vi "Calibration.vi"(2 "Analogue In":refnum<k21>, 3 "Digital In":refnum<k21>) -> (0 "Analogue In Out":refnum<k21>, 1 "Digital Out":refnum<k21>)   [LabVIEW 2015]
uses:
  CalibrationEnum.ctl
  <vilib>/DAQmx/write.llb/DAQmx Write (Digital 1D Bool NChan 1Samp 1Line).vi
  <vilib>/DAQmx/write.llb/DAQmx Write (Analog 1D DBL NChan 1Samp).vi
  GlobalVariables.vi
  <vilib>/DAQmx/create/channels.llb/DAQmx Create Channel (AO-Voltage-Basic).vi
  <vilib>/DAQmx/create/channels.llb/DAQmx Create Channel (DO-Digital Output).vi
  <vilib>/DAQmx/miscellaneous.llb/DAQmx Fill In Error Info.vi
  <resource>/objmgr/daqmx.rc
panel:
  in  "Listbox":i32(listbox)
  in  "Calibration Coordinates":T1
  in  "Calibration Map":T2
  in  "Piezo Focus /um":dbl(slide)=5.0 scale=0.0..10.0
  out "Enum":T3=enum."YMirrorVolt"
  in  "stop":bool
  in  "Z Voltage /V":dbl(slide)=-3.815028901734104 scale=-10.0..10.0
  in  "Y Voltage /V":dbl(slide)=2.485549132947977 scale=-10.0..10.0
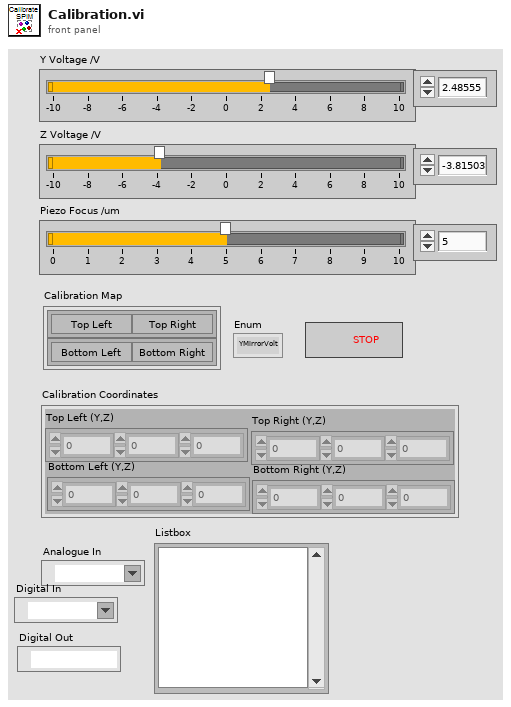
[diagram p1: front panel]
types:
  T1 = cluster{"Top Left (Y,Z)":dbl[], "Top Right (Y,Z)":dbl[], "Bottom Left (Y,Z)":dbl[], "Bottom Right (Y,Z)":dbl[]}
  T2 = cluster{"Cluster 2":cluster{"Top Left":bool, "Top Right":bool}, "Cluster":cluster{"Bottom Left":bool, "Bottom Right":bool}}
  T3 = typedef "CalibrationEnum.ctl" = enum16{"PiezoVolt", "YMirrorVolt", "ZMirrorVolt", "idle"}
  T4 = cluster{dbl[], "Top Right (Y,Z)":dbl[], "Bottom Left (Y,Z)":dbl[], "Bottom Right (Y,Z)":dbl[]}
  T5 = cluster{"Top Left (Y,Z)":dbl[], dbl[], "Bottom Left (Y,Z)":dbl[], "Bottom Right (Y,Z)":dbl[]}
  T6 = cluster{"Top Left (Y,Z)":dbl[], "Top Right (Y,Z)":dbl[], dbl[], "Bottom Right (Y,Z)":dbl[]}
  T7 = cluster{"Top Left (Y,Z)":dbl[], "Top Right (Y,Z)":dbl[], "Bottom Left (Y,Z)":dbl[], dbl[]}
  T8 = cluster{"Top Left":dbl[], "Top Right":dbl[], "Bottom Left":dbl[], "Bottom Right":dbl[]}
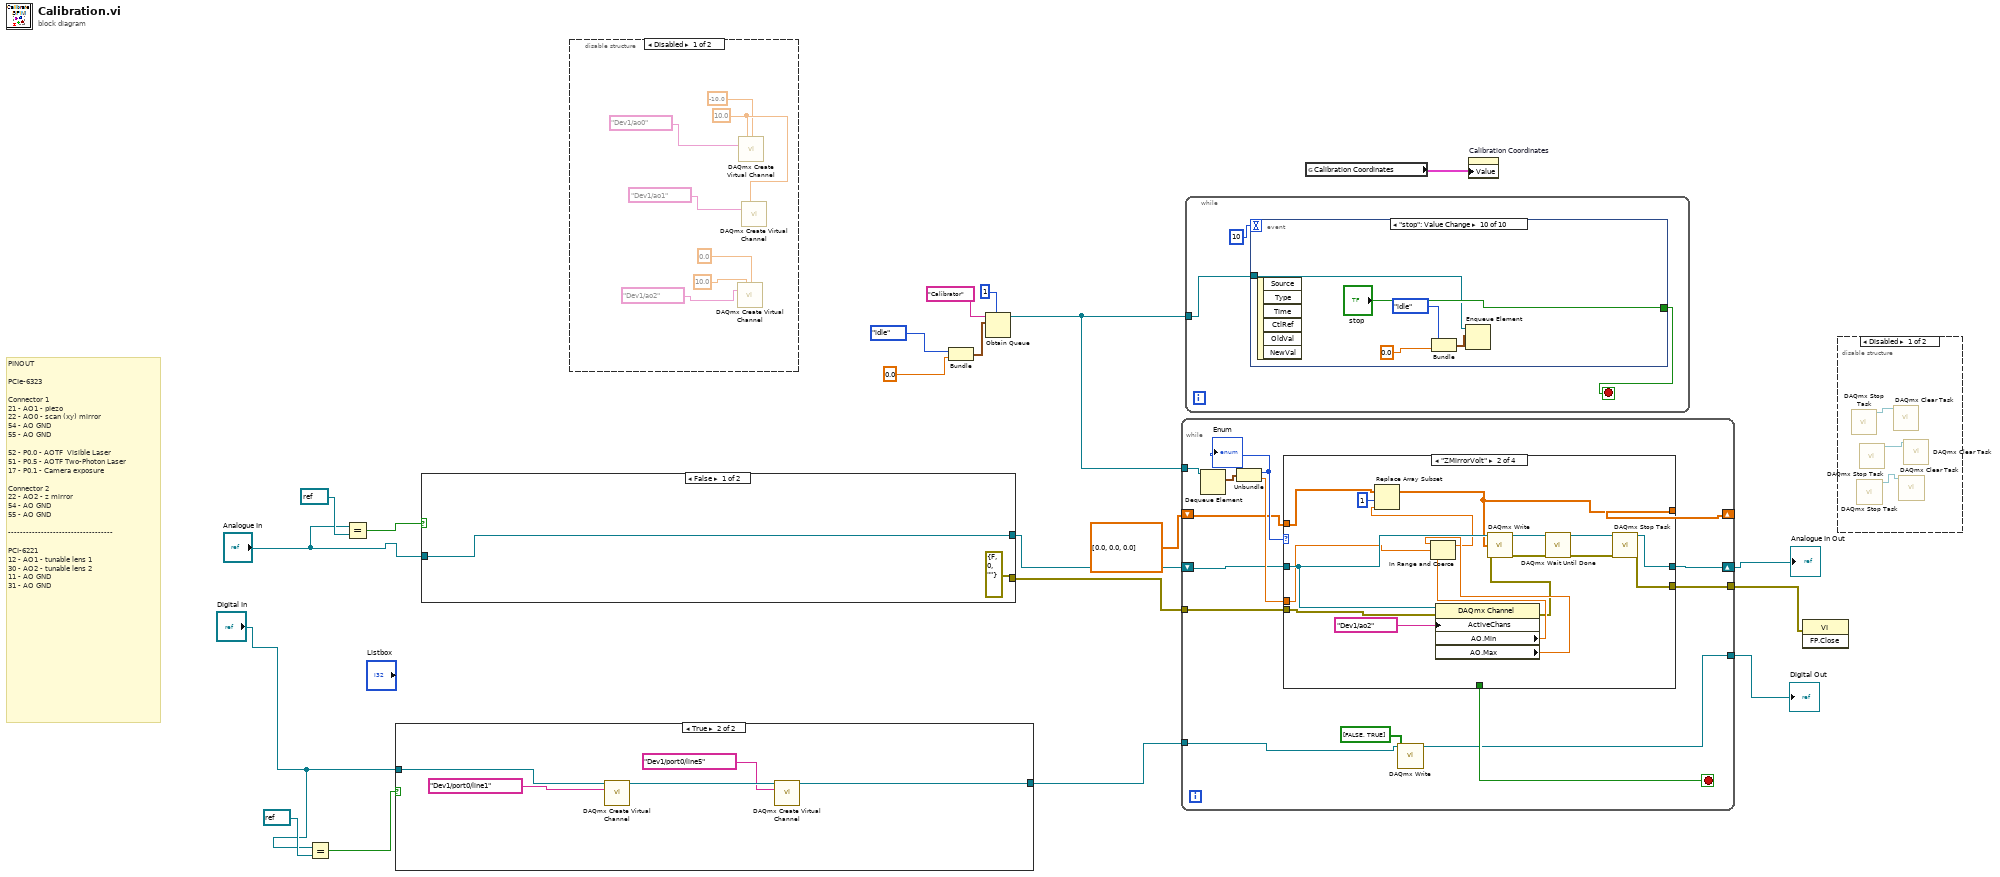
[diagram p0: block diagram]
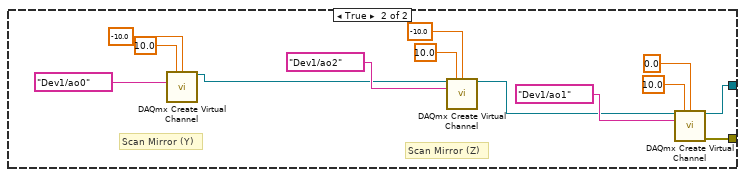
[diagram p3: hidden frame]
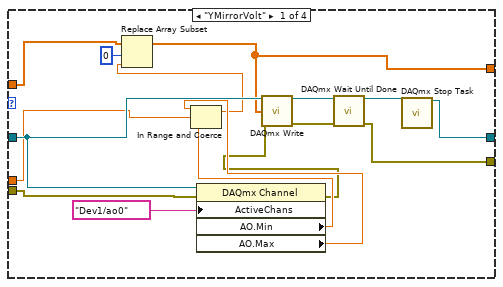
[diagram p6: hidden frame]
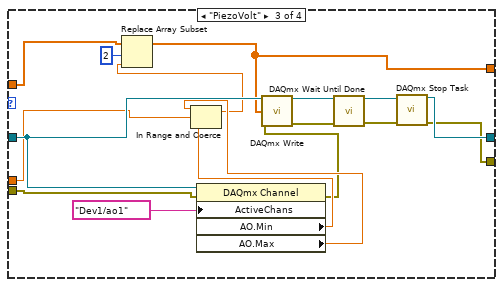
[diagram p7: hidden frame]
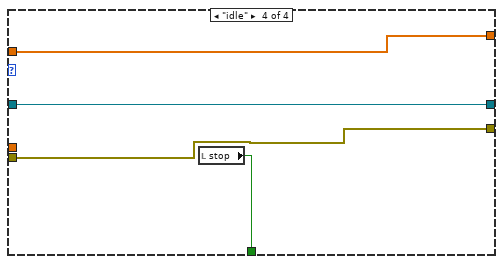
[diagram p8: hidden frame]
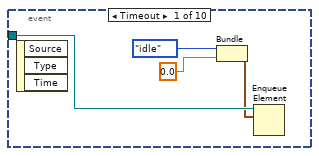
[diagram p9: hidden frame]
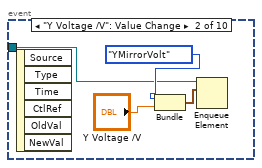
[diagram p10: hidden frame]
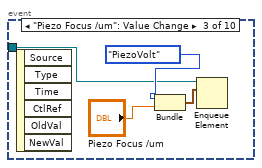
[diagram p11: hidden frame]
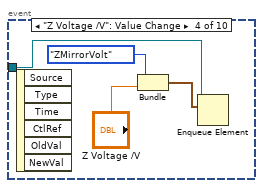
[diagram p12: hidden frame]
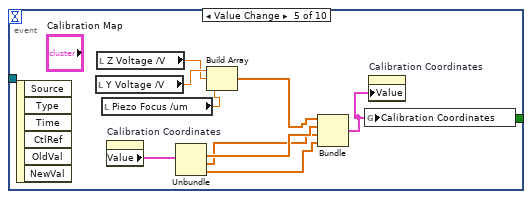
[diagram p13: hidden frame]
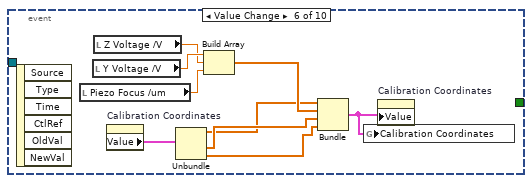
[diagram p14: hidden frame]
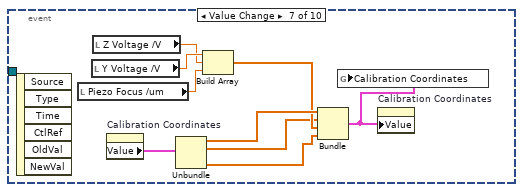
[diagram p15: hidden frame]
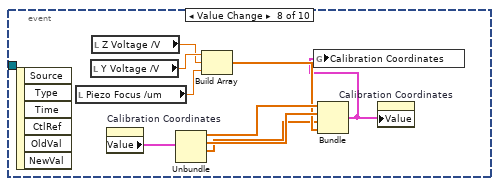
[diagram p16: hidden frame]
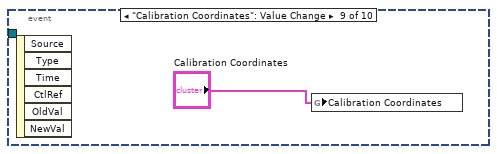
[diagram p17: hidden frame]
diagram:
  # "PINOUT\n\nPCIe-6323\n\nConnector 1\n21 - AO1 - piezo\n22 - AO0 - scan (xy) mirror\n54 - AO GND\n55 - AO GND\n\n52 - P0.0 - AOTF  Visible Laser\n51 - P0.5 - AOTF Two-Photon Laser\n17 - P0.1 - Camera exposure\n\nConnector 2\n22 - AO2 - z mirror\n54 - AO GND\n55 - AO GND\n\n-----------------------------------\n\nPCI-6221\n12 - AO1 - tunable lens 1\n30 - AO2 - tunable lens 2\n11 - AO GND\n31 - AO GND"
  n1 = Equal?(x="Digital In", y=refnum<k21> refnum ("Mirror Y")) -> (x = y?=w2:bool)
  n2 = Equal?(x="Analogue In", y=refnum<k21> refnum ("Mirror Y")) -> (x = y?=w12:bool)
  n3 = case shown="True" w2 {
    tunnel: "Digital In" -> [w21 w23]
    tunnel: [w21 w22] -> w1
    frame False {
    }
    frame True {
      n4 = call-poly <vilib>:"DAQmx Create Virtual Channel.vi"("task in"=w23, "lines"=tag "Dev1/port0/line1") -> ("task out"=w26:refnum<k21>)  [unwired: 12 in, 1 out]
      n5 = call-poly <vilib>:"DAQmx Create Virtual Channel.vi"("task in"=w26, "lines"=tag "Dev1/port0/line5") -> ("task out"=w22:refnum<k21>)  [unwired: 12 in, 1 out]
    }
  }
  n6 = case shown="False" w12 {
    tunnel: [w28 w31] -> w9
    tunnel: "Analogue In" -> [w28 _]
    tunnel: [errorcluster {"status"=FALSE, "code"=0, "source"=""} ("error out") w29] -> w6
    frame False {
    }
    frame True {
      # "Scan Mirror (Z)"
      # "Scan Mirror (Y)"
      n7 = call-poly <vilib>:"DAQmx Create Virtual Channel.vi"("maximum value"=10.0, "minimum value"=-10.0, "physical channels"=tag "Dev1/ao0") -> ("task out"=w36:refnum<k21>)  [unwired: 11 in, 1 out]
      n8 = call-poly <vilib>:"DAQmx Create Virtual Channel.vi"("task in"=w36, "maximum value"=10.0, "minimum value"=-10.0, "physical channels"=tag "Dev1/ao2") -> ("task out"=w32:refnum<k21>)  [unwired: 10 in, 1 out]
      n9 = call-poly <vilib>:"DAQmx Create Virtual Channel.vi"("task in"=w32, "maximum value"=10.0, "minimum value"=0.0, "physical channels"=tag "Dev1/ao1") -> ("task out"=w31:refnum<k21>, "error out"=w29:errorcluster)  [unwired: 10 in]
    }
  }
  n10 = disable-structure shown="Disabled" {
    frame Disabled {
      w48 = 10.0 ("maximum value")
      n11 = call-poly <vilib>:"DAQmx Create Virtual Channel.vi"("maximum value"=10.0 ("minimum value"), "minimum value"=0.0 ("maximum value"), "physical channels"=tag "Dev1/ao2") -> ()  [unwired: 11 in, 2 out]
      n12 = call-poly <vilib>:"DAQmx Create Virtual Channel.vi"("maximum value"=w48, "minimum value"=-10.0, "physical channels"=tag "Dev1/ao0") -> ()  [unwired: 11 in, 2 out]
      n13 = call-poly <vilib>:"DAQmx Create Virtual Channel.vi"("maximum value"=w48, "physical channels"=tag "Dev1/ao1") -> ()  [unwired: 12 in, 2 out]
    }
    frame Enabled {
    }
  }
  n14 = Bundle(CalibrationEnum."idle", 0.0) -> (w15:cluster{T3, dbl})  [unwired: 1 in]
  n15 = Obtain Queue(max queue size (-1, unlimited)=1, name (unnamed)="Calibrator", element data type=w15) -> (queue out=w20:refnum<queue>)  [unwired: 2 in, 2 out]
  n16 = while {
    tunnel: w20 -> [w62]
    shift-right: [w58] -> w10
    shift-left: w9 -> [w59]
    shift-right: [w54] -> _
    shift-left: dbl[] [0.0, 0.0, 0.0] -> [w55]
    tunnel: [w52] -> w7
    tunnel: w6 -> [w53]
    tunnel: [w49] -> w5
    tunnel: w1 -> [w51]
    stop <- w57 stop-if-true
    n17 = Dequeue Element(queue=w62) -> (element=w61:cluster{T3, dbl})  [unwired: 2 in, 3 out]
    n18 = Unbundle(w61) -> (w56:T3, w60:dbl)
    "Enum" <- w56
    n19 = case shown="\"ZMirrorVolt\"" w56 {
      tunnel: w60 -> [w73 w90 w107 _]
      tunnel: w59 -> [w76 w93 w110 w116]
      tunnel: [w66 w83 w100 w116] -> w58
      tunnel: [_ _ _ w115] -> w57
      tunnel: w55 -> [w71 w88 w105 w114]
      tunnel: [w69 w86 w103 w114] -> w54
      tunnel: w53 -> [w63 w80 w97 w113]
      tunnel: [w65 w81 w99 w113] -> w52
      frame "YMirrorVolt" {
        n20 = property class="DAQmx Channel"(reference=w76, error in=w63, "ActiveChans"=tag "Dev1/ao0") -> (error out=w64:errorcluster, "AO.Min"=w75:dbl, "AO.Max"=w74:dbl)  [unwired: 1 out]
        n21 = In Range and Coerce(upper limit=w74, x=w73, lower limit=w75) -> (coerced(x)=w70:dbl)  [unwired: 1 out]
        n22 = Replace Array Subset(array=w71, new element=w70, index=0) -> (w69:dbl[])
        n23 = call-poly <vilib>:"DAQmx Write.vi"("task/channels in"=w76, "data"=w69, "error in"=w64) -> ("task out"=w78:refnum<k21>, "error out"=w68:errorcluster)  [unwired: 10 in, 1 out]
        n24 = call <vilib>:"DAQmx Wait Until Done.vi"("task/channels in"=w78, "error in"=w68) -> ("task out"=w67:refnum<k21>, "error out"=w65:errorcluster)  [unwired: 12 in]
        n25 = call <vilib>:"DAQmx Stop Task.vi"("task/channels in"=w67) -> ("task out"=w66:refnum<k21>)  [unwired: 13 in, 1 out]
      }
      frame "ZMirrorVolt" {
        n26 = property class="DAQmx Channel"(reference=w93, error in=w80, "ActiveChans"=tag "Dev1/ao2") -> (error out=w79:errorcluster, "AO.Min"=w92:dbl, "AO.Max"=w91:dbl)  [unwired: 1 out]
        n27 = In Range and Coerce(upper limit=w91, x=w90, lower limit=w92) -> (coerced(x)=w87:dbl)  [unwired: 1 out]
        n28 = Replace Array Subset(array=w88, new element=w87, index=1) -> (w86:dbl[])
        n29 = call-poly <vilib>:"DAQmx Write.vi"("task/channels in"=w93, "data"=w86, "error in"=w79) -> ("task out"=w95:refnum<k21>, "error out"=w85:errorcluster)  [unwired: 10 in, 1 out]
        n30 = call <vilib>:"DAQmx Wait Until Done.vi"("task/channels in"=w95, "error in"=w85) -> ("task out"=w84:refnum<k21>, "error out"=w82:errorcluster)  [unwired: 12 in]
        n31 = call <vilib>:"DAQmx Stop Task.vi"("task/channels in"=w84, "error in"=w82) -> ("task out"=w83:refnum<k21>, "error out"=w81:errorcluster)  [unwired: 12 in]
      }
      frame "PiezoVolt" {
        n32 = property class="DAQmx Channel"(reference=w110, error in=w97, "ActiveChans"=tag "Dev1/ao1") -> (error out=w96:errorcluster, "AO.Min"=w109:dbl, "AO.Max"=w108:dbl)  [unwired: 1 out]
        n33 = In Range and Coerce(upper limit=w108, x=w107, lower limit=w109) -> (coerced(x)=w104:dbl)  [unwired: 1 out]
        n34 = Replace Array Subset(array=w105, new element=w104, index=2) -> (w103:dbl[])
        n35 = call-poly <vilib>:"DAQmx Write.vi"("task/channels in"=w110, "data"=w103, "error in"=w96) -> ("task out"=w112:refnum<k21>, "error out"=w98:errorcluster)  [unwired: 10 in, 1 out]
        n36 = call <vilib>:"DAQmx Wait Until Done.vi"("task/channels in"=w112, "error in"=w98) -> ("task out"=w102:refnum<k21>, "error out"=w101:errorcluster)  [unwired: 12 in]
        n37 = call <vilib>:"DAQmx Stop Task.vi"("task/channels in"=w102, "error in"=w101) -> ("task out"=w100:refnum<k21>, "error out"=w99:errorcluster)  [unwired: 12 in]
      }
      frame "idle" {
        n38 = local read "stop"() -> (w115:bool)
      }
    }
    n39 = call-poly <vilib>:"DAQmx Write.vi"("task/channels in"=w51, "data"=bool[] [FALSE, TRUE]) -> ("task out"=w49:refnum<k21>)  [unwired: 11 in, 2 out]
  }
  "Analogue In Out" <- w10
  "Digital Out" <- w5
  n40 = while {
    tunnel: w20 -> [w117]
    stop <- w118 stop-if-true
    n41 = event shown="[9] \"stop\": Value Change" {
      selector: _ -> [_ _ _ _ _ _ _ _ _ _]
      dyn-events: _ -> [_ _ _ _ _ _ _ _ _ _]
      timeout: 10 -> [_ _ _ _ _ _ _ _ _ _]
      tunnel: [_ _ _ _ _ _ _ _ _ "stop"] -> w118
      tunnel: w117 -> [w121 w124 w129 w132 _ _ _ _ _ w176]
      event Timeout {
        n42 = event-data() -> ()  [unwired: 1 in, 3 out]
        n43 = Bundle(CalibrationEnum."idle", "minimum value"=0.0) -> (w120:cluster{T3, "minimum value":dbl})  [unwired: 1 in]
        n44 = Enqueue Element(queue=w121, element=w120) -> ()  [unwired: 2 in, 3 out]
      }
      event "Y Voltage /V": Value Change {
        n45 = event-data() -> ()  [unwired: 1 in, 6 out]
        n46 = Bundle(CalibrationEnum."YMirrorVolt", "Y Voltage /V"="Y Voltage /V") -> (w125:cluster{T3, "Y Voltage /V":dbl})  [unwired: 1 in]
        n47 = Enqueue Element(queue=w124, element=w125) -> ()  [unwired: 2 in, 3 out]
      }
      event "Piezo Focus /um": Value Change {
        n48 = event-data() -> ()  [unwired: 1 in, 6 out]
        n49 = Bundle(CalibrationEnum."PiezoVolt", "Piezo Focus /um"="Piezo Focus /um") -> (w130:cluster{T3, "Piezo Focus /um":dbl})  [unwired: 1 in]
        n50 = Enqueue Element(queue=w129, element=w130) -> ()  [unwired: 2 in, 3 out]
      }
      event "Z Voltage /V": Value Change {
        n51 = event-data() -> ()  [unwired: 1 in, 6 out]
        n52 = Bundle(CalibrationEnum."ZMirrorVolt", "Z Voltage /V"="Z Voltage /V") -> (w133:cluster{T3, "Z Voltage /V":dbl})  [unwired: 1 in]
        n53 = Enqueue Element(queue=w132, element=w133) -> ()  [unwired: 2 in, 3 out]
      }
      event "Calibration Map.Cluster 2.Top Left": Value Change {
        n54 = event-data() -> ()  [unwired: 1 in, 6 out]
        n55 = local read "Y Voltage /V"() -> (w143:dbl)
        n56 = local read "Z Voltage /V"() -> (w142:dbl)
        n57 = local read "Piezo Focus /um"() -> (w136:dbl)
        n58 = property on="Calibration Coordinates" class="Clust (strict)"() -> ("Value"=w144:T1)  [unwired: 2 in, 2 out]
        n59 = Unbundle(w144) -> ("Top Right (Y,Z)"=w140:dbl[], "Bottom Left (Y,Z)"=w139:dbl[], "Bottom Right (Y,Z)"=w138:dbl[])  [unwired: 1 out]
        n60 = Build Array(w143, w142, w136) -> (w141:dbl[])
        n61 = Bundle(w141, "Top Right (Y,Z)"=w140, "Bottom Left (Y,Z)"=w139, "Bottom Right (Y,Z)"=w138) -> (w137:T4)  [unwired: 1 in]
        n62 = global write "GlobalVariables.vi" "Calibration Coordinates"(w137) -> ()
        n63 = property on="Calibration Coordinates" class="Clust (strict)"("Value"=w137) -> ()  [unwired: 2 in, 2 out]
      }
      event "Calibration Map.Cluster 2.Top Right": Value Change {
        n64 = event-data() -> ()  [unwired: 1 in, 6 out]
        n65 = local read "Piezo Focus /um"() -> (w145:dbl)
        n66 = local read "Y Voltage /V"() -> (w152:dbl)
        n67 = local read "Z Voltage /V"() -> (w151:dbl)
        n68 = property on="Calibration Coordinates" class="Clust (strict)"() -> ("Value"=w153:T1)  [unwired: 2 in, 2 out]
        n69 = Unbundle(w153) -> ("Top Left (Y,Z)"=w147:dbl[], "Bottom Left (Y,Z)"=w150:dbl[], "Bottom Right (Y,Z)"=w149:dbl[])  [unwired: 1 out]
        n70 = Build Array(w152, w151, w145) -> (w148:dbl[])
        n71 = Bundle("Top Left (Y,Z)"=w147, w148, "Bottom Left (Y,Z)"=w150, "Bottom Right (Y,Z)"=w149) -> (w146:T5)  [unwired: 1 in]
        n72 = global write "GlobalVariables.vi" "Calibration Coordinates"(w146) -> ()
        n73 = property on="Calibration Coordinates" class="Clust (strict)"("Value"=w146) -> ()  [unwired: 2 in, 2 out]
      }
      event "Calibration Map.Cluster.Bottom Left": Value Change {
        n74 = event-data() -> ()  [unwired: 1 in, 6 out]
        n75 = local read "Piezo Focus /um"() -> (w154:dbl)
        n76 = local read "Y Voltage /V"() -> (w161:dbl)
        n77 = local read "Z Voltage /V"() -> (w160:dbl)
        n78 = property on="Calibration Coordinates" class="Clust (strict)"() -> ("Value"=w162:T1)  [unwired: 2 in, 2 out]
        n79 = Unbundle(w162) -> ("Top Left (Y,Z)"=w158:dbl[], "Top Right (Y,Z)"=w156:dbl[], "Bottom Right (Y,Z)"=w159:dbl[])  [unwired: 1 out]
        n80 = Build Array(w161, w160, w154) -> (w157:dbl[])
        n81 = Bundle("Top Left (Y,Z)"=w158, "Top Right (Y,Z)"=w156, w157, "Bottom Right (Y,Z)"=w159) -> (w155:T6)  [unwired: 1 in]
        n82 = global write "GlobalVariables.vi" "Calibration Coordinates"(w155) -> ()
        n83 = property on="Calibration Coordinates" class="Clust (strict)"("Value"=w155) -> ()  [unwired: 2 in, 2 out]
      }
      event "Calibration Map.Cluster.Bottom Right": Value Change {
        n84 = event-data() -> ()  [unwired: 1 in, 6 out]
        n85 = local read "Piezo Focus /um"() -> (w163:dbl)
        n86 = local read "Y Voltage /V"() -> (w170:dbl)
        n87 = local read "Z Voltage /V"() -> (w169:dbl)
        n88 = property on="Calibration Coordinates" class="Clust (strict)"() -> ("Value"=w171:T1)  [unwired: 2 in, 2 out]
        n89 = Unbundle(w171) -> ("Top Left (Y,Z)"=w168:dbl[], "Top Right (Y,Z)"=w167:dbl[], "Bottom Left (Y,Z)"=w165:dbl[])  [unwired: 1 out]
        n90 = Build Array(w170, w169, w163) -> (w166:dbl[])
        n91 = Bundle("Top Left (Y,Z)"=w168, "Top Right (Y,Z)"=w167, "Bottom Left (Y,Z)"=w165, w166) -> (w164:T7)  [unwired: 1 in]
        n92 = global write "GlobalVariables.vi" "Calibration Coordinates"(w164) -> ()
        n93 = property on="Calibration Coordinates" class="Clust (strict)"("Value"=w164) -> ()  [unwired: 2 in, 2 out]
      }
      event "Calibration Coordinates": Value Change {
        n94 = event-data() -> ()  [unwired: 1 in, 6 out]
        n95 = global write "GlobalVariables.vi" "Calibration Coordinates"("Calibration Coordinates") -> ()
      }
      event "stop": Value Change {
        n96 = event-data() -> ()  [unwired: 1 in, 6 out]
        n97 = Bundle(CalibrationEnum."idle", "minimum value"=0.0) -> (w173:cluster{T3, "minimum value":dbl})  [unwired: 1 in]
        n98 = Enqueue Element(queue=w176, element=w173) -> ()  [unwired: 2 in, 3 out]
      }
    }
  }
  n99 = global read "GlobalVariables.vi" "Calibration Coordinates"() -> (w14:T8)
  n100 = property on="Calibration Coordinates" class="Clust (strict)"("Value"=w14) -> ()  [unwired: 2 in, 2 out]
  n101 = invoke class="VI" method="FP.Close"(error in=w7) -> ()  [unwired: 2 in, 3 out]
  n102 = disable-structure shown="Disabled" {
    frame Disabled {
      n103 = call <vilib>:"DAQmx Stop Task.vi"() -> ("task out"=w180:refnum<k21>)  [unwired: 14 in, 1 out]
      n104 = call <vilib>:"DAQmx Stop Task.vi"() -> ("task out"=w178:refnum<k21>)  [unwired: 14 in, 1 out]
      n105 = call <vilib>:"DAQmx Stop Task.vi"() -> ("task out"=w179:refnum<k21>)  [unwired: 14 in, 1 out]
      n106 = call <vilib>:"DAQmx Clear Task.vi"("task in"=w180) -> ()  [unwired: 14 in, 1 out]
      n107 = call <vilib>:"DAQmx Clear Task.vi"("task in"=w178) -> ()  [unwired: 14 in, 1 out]
      n108 = call <vilib>:"DAQmx Clear Task.vi"("task in"=w179) -> ()  [unwired: 14 in, 1 out]
    }
    frame Enabled {
    }
  }
